vi "MedConfig.vi"(8 "error in (no error)":errorcluster, 11 "Array Parsed Expression":T2[](array[typedef])) -> (0 "error out":errorcluster, 3 "Array Parsed Expression Out":T2[](array[typedef]))   [LabVIEW 2014, in "MathProg.lvlib"]
doc: "Configura las Mediciones."
uses:
  MathProg.lvlib
  TypeDefs/ParsedExpression.ctl
  TypeDefs/typeMed.ctl
panel:
  in  "Resultado:":T1
  out "Tol. Inf. Abs:":sgl
  out "Pre. TI Abs:":sgl
  out "Pre. TS Abs:":sgl
  out "Tol. Sup. Abs:":sgl
  in  "Tol. Inf.:":sgl max=0
  in  "Pre. TI:":sgl max=0
  in  "Pre. TS:":sgl min=0
  in  "Tol. Sup.:":sgl min=0
  in  "Nominal:":sgl
  in  "Description":string caption="Descripción:"
  in  "Stop Med":bool
  in  "Delete Med":bool
  in  "Add Med":bool
  in  "Mediciones":i32(listbox)=-1
  in  "Cancel Med":bool
  in  "Save Med":bool
  in  "Formula:":string
  in  "Edit Med":bool
  out "Medición:":string="M1"
  # "Val Absolutos"
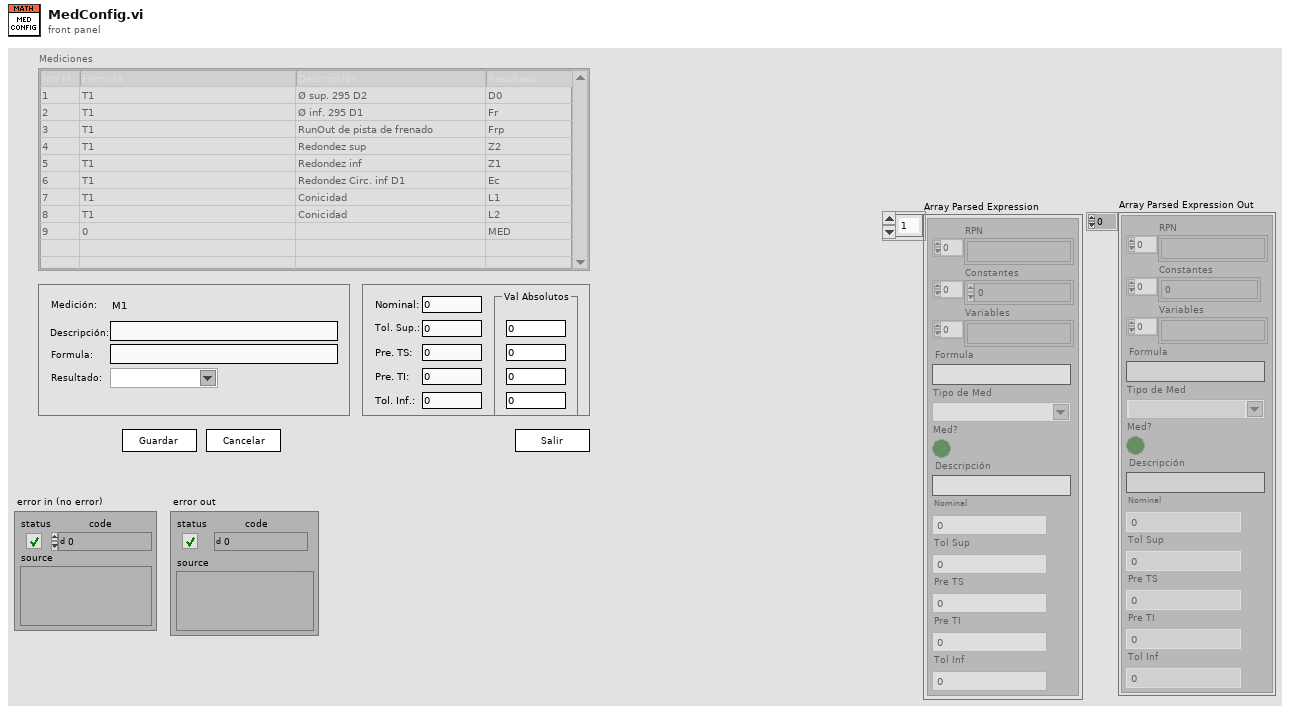
[diagram p1: front panel]
types:
  T1 = typedef "MathProg.lvlib/typeMed.ctl" = string
  T2 = typedef "MathProg.lvlib/ParsedExpression.ctl" = cluster{"RPN ":string[], "Constantes":sgl[], "Variables":string[], "Formula":string, "Tipo de Med":T1, "Med?":bool, "Descripción":string, "Nominal":sgl, "Tol Sup":sgl, "Pre TS":sgl, "Pre TI":sgl, "Tol Inf":sgl}
  T3 = enum8{"Enabled", "Disabled", "Disabled and Grayed Out"}
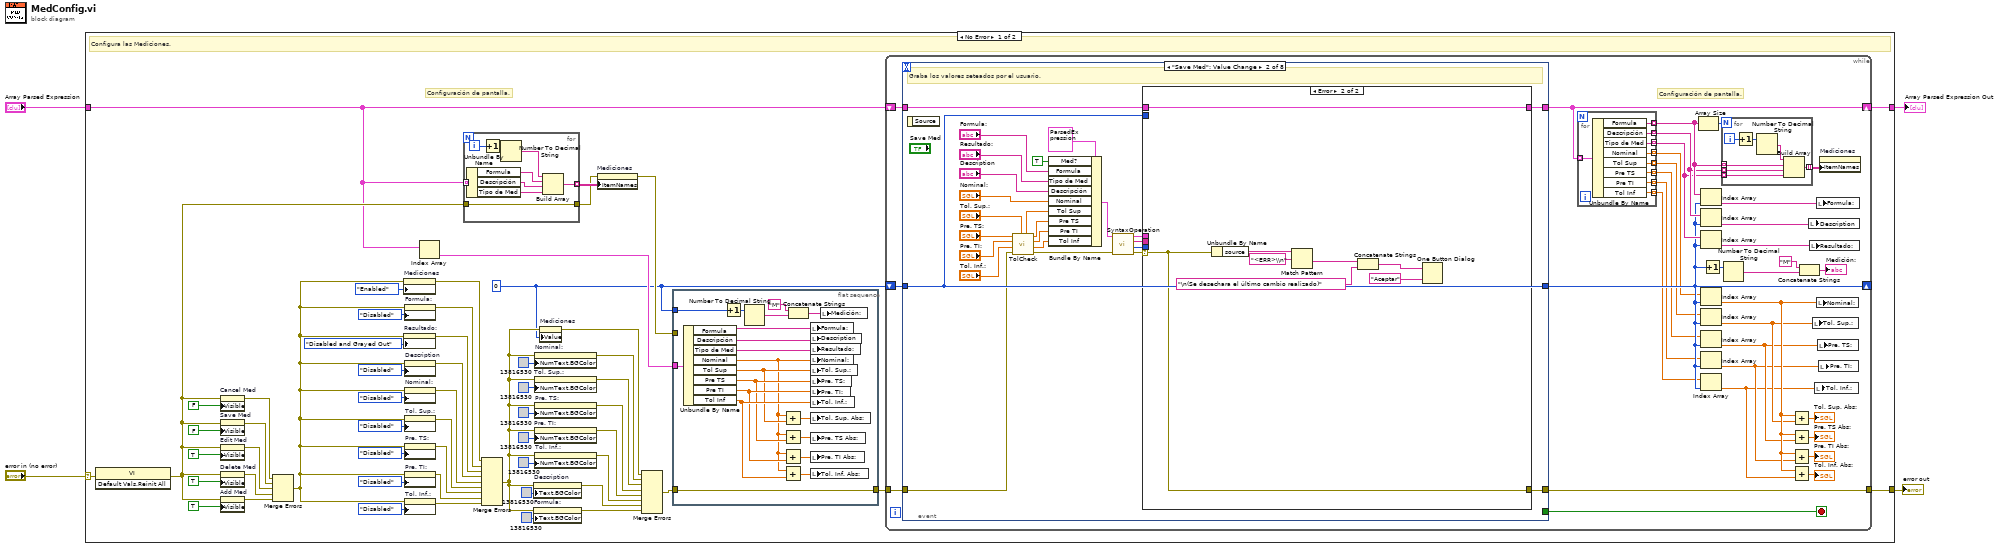
[diagram p0: block diagram]
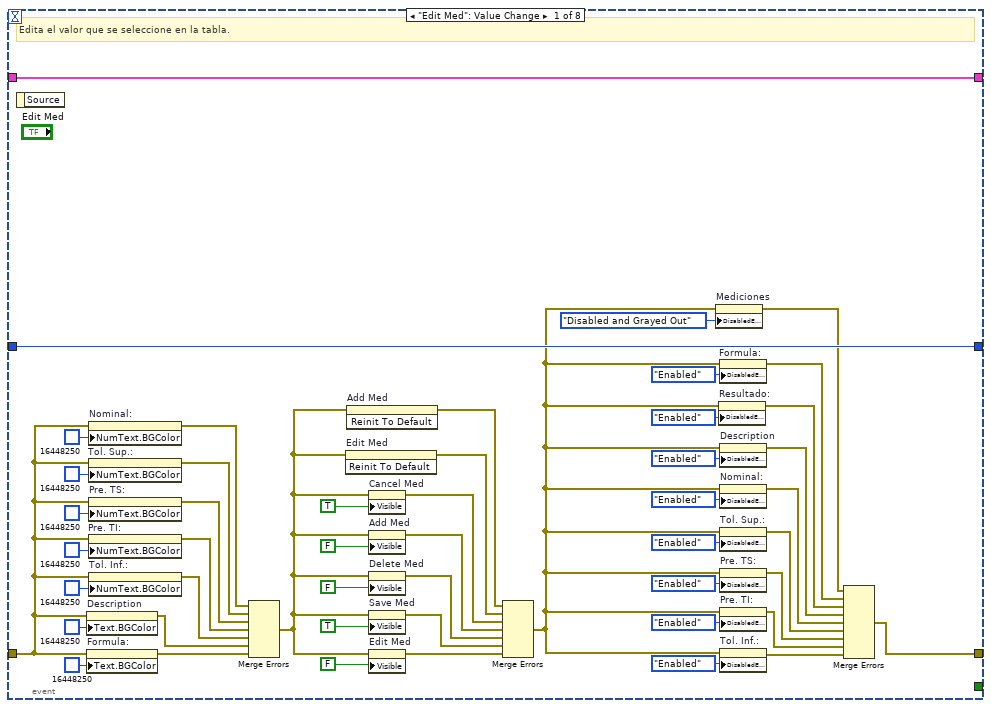
[diagram p2: hidden frame]
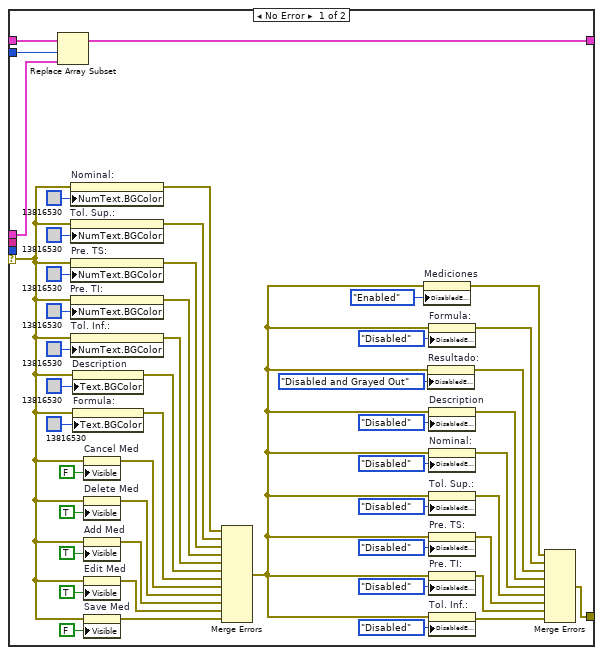
[diagram p3: hidden frame]
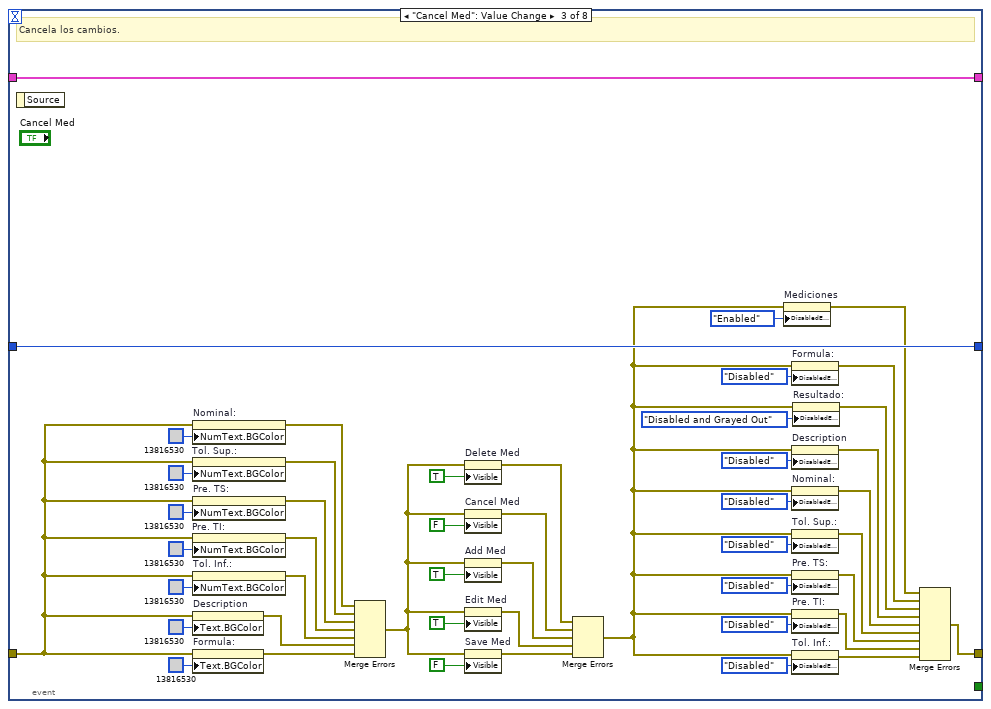
[diagram p4: hidden frame]
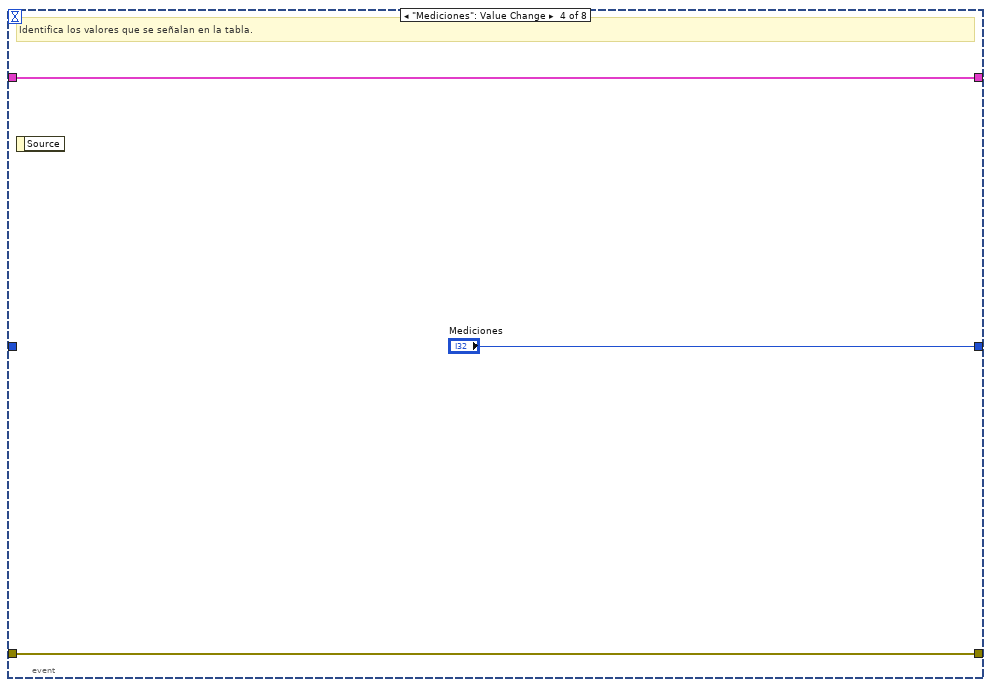
[diagram p5: hidden frame]
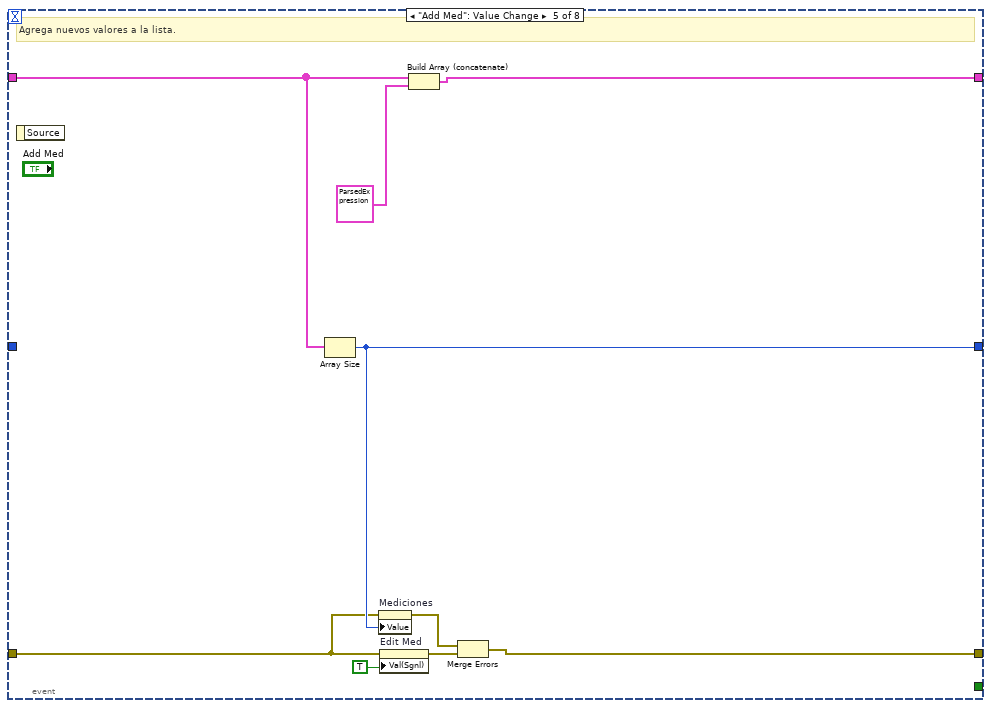
[diagram p6: hidden frame]
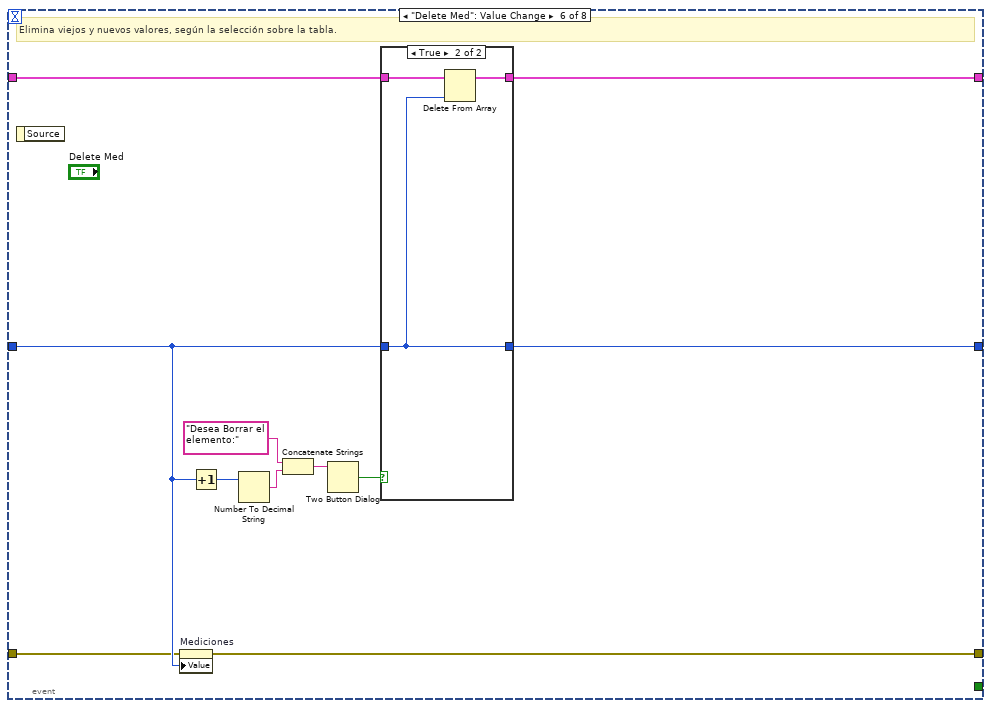
[diagram p7: hidden frame]
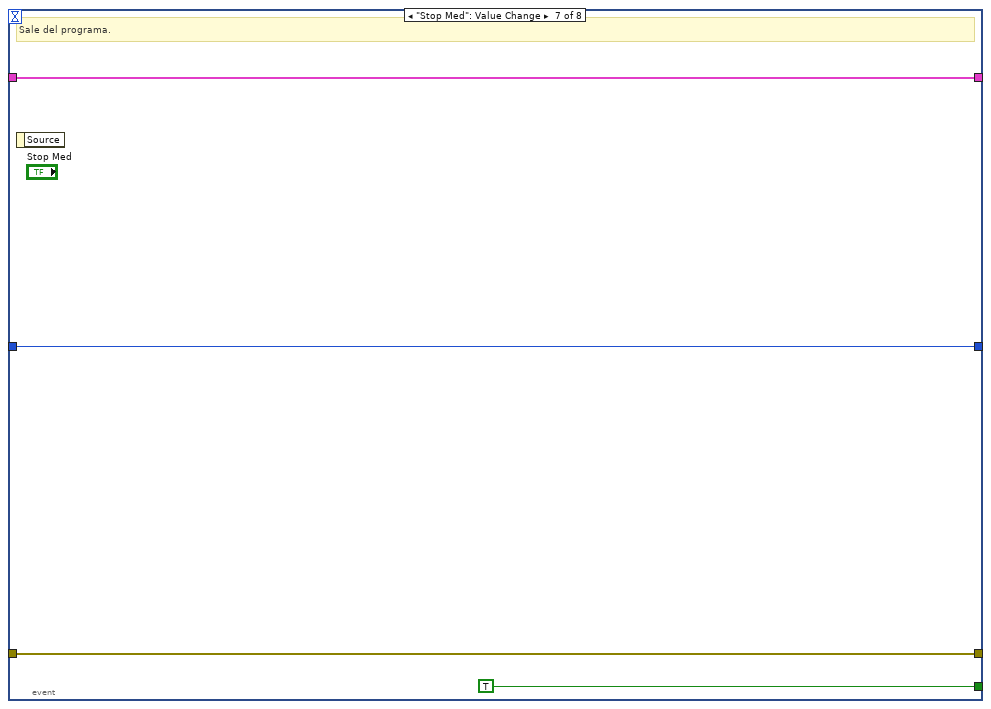
[diagram p9: hidden frame]
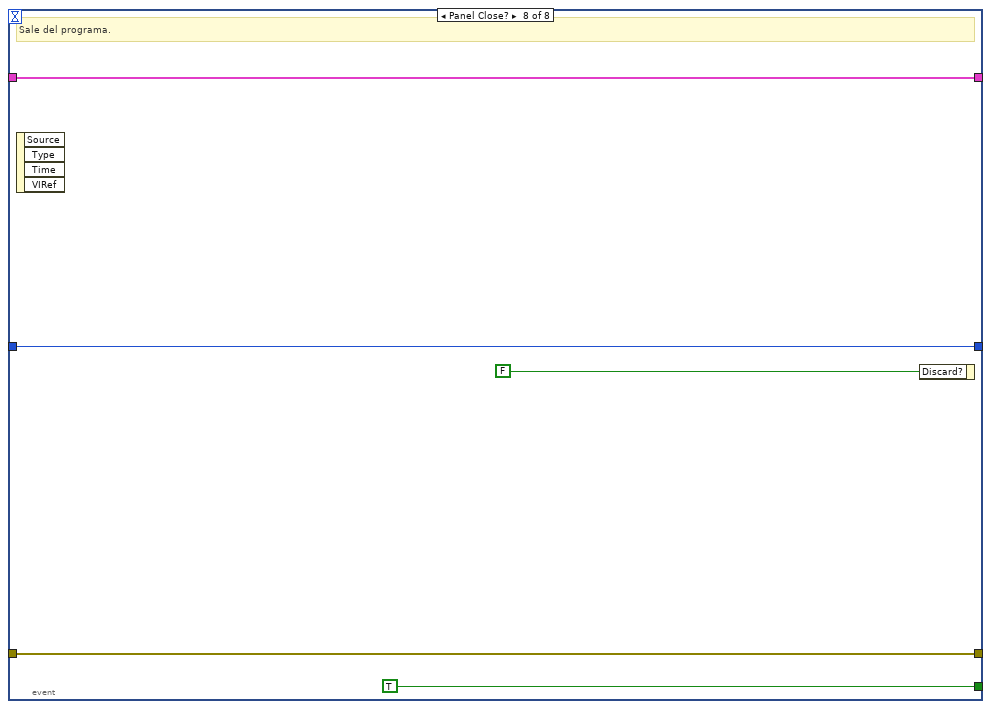
[diagram p10: hidden frame]
diagram:
  n1 = case shown="No Error" "error in (no error)" {
    selector: "error in (no error)" -> [w9 w356]
    tunnel: [w61 w356] -> w4
    tunnel: [w37 w357] -> w3
    tunnel: "Array Parsed Expression" -> [w19 w357]
    frame No Error {
      w12 = 0 ("disabled index (col)")
      # "Configuración de pantalla."
      # "Configura las Mediciones."
      n2 = invoke class="VI" method="Default Vals.Reinit All"(error in=w9) -> (error out=w36:errorcluster)  [unwired: 2 in, 2 out]
      n3 = property on="Cancel Med" class="Bool"(error in=w36, "Visible"=FALSE) -> (error out=w54:errorcluster)  [unwired: 1 in, 1 out]
      n4 = property on="Save Med" class="Bool"(error in=w36, "Visible"=FALSE) -> (error out=w58:errorcluster)  [unwired: 1 in, 1 out]
      n5 = property on="Edit Med" class="Bool (strict)"(error in=w36, "Visible"=TRUE) -> (error out=w57:errorcluster)  [unwired: 1 in, 1 out]
      n6 = property on="Delete Med" class="Bool"(error in=w36, "Visible"=TRUE) -> (error out=w52:errorcluster)  [unwired: 1 in, 1 out]
      n7 = property on="Add Med" class="Bool (strict)"(error in=w36, "Visible"=TRUE) -> (error out=w50:errorcluster)  [unwired: 1 in, 1 out]
      n8 = Merge Errors(w54, w58, w57, w52, w50) -> (w6:errorcluster)
      n9 = property on="Mediciones" class="MCListbox (strict)"(error in=w6, "DisabledEnum"=T3."Enabled" ("Disabled")) -> (error out=w10:errorcluster)  [unwired: 1 in, 1 out]
      n10 = property on="Resultado:" class="CmbBox (strict)"(error in=w6, "DisabledEnum"=T3."Disabled and Grayed Out" ("Disabled")) -> (error out=w7:errorcluster)  [unwired: 1 in, 1 out]
      n11 = property on="Formula:" class="Str"(error in=w6, "DisabledEnum"=T3."Disabled" ("Disabled")) -> (error out=w35:errorcluster)  [unwired: 1 in, 1 out]
      n12 = property on="Description" class="Str"(error in=w6, "DisabledEnum"=T3."Disabled" ("Disabled")) -> (error out=w34:errorcluster)  [unwired: 1 in, 1 out]
      n13 = property on="Nominal:" class="DigNum (strict)"(error in=w6, "DisabledEnum"=T3."Disabled" ("Disabled")) -> (error out=w33:errorcluster)  [unwired: 1 in, 1 out]
      n14 = property on="Tol. Sup.:" class="DigNum (strict)"(error in=w6, "DisabledEnum"=T3."Disabled" ("Disabled")) -> (error out=w32:errorcluster)  [unwired: 1 in, 1 out]
      n15 = property on="Pre. TS:" class="DigNum (strict)"(error in=w6, "DisabledEnum"=T3."Disabled" ("Disabled")) -> (error out=w31:errorcluster)  [unwired: 1 in, 1 out]
      n16 = property on="Pre. TI:" class="DigNum (strict)"(error in=w6, "DisabledEnum"=T3."Disabled" ("Disabled")) -> (error out=w30:errorcluster)  [unwired: 1 in, 1 out]
      n17 = property on="Tol. Inf.:" class="DigNum (strict)"(error in=w6, "DisabledEnum"=T3."Disabled" ("Disabled")) -> (error out=w24:errorcluster)  [unwired: 1 in, 1 out]
      n18 = Index Array(array=w19) -> (element=w18:T2)  [unwired: 1 in]
      n19 = for {
        tunnel: w19 -> [w89] mode=indexing
        tunnel: w36 -> [w81]
        tunnel: [w82] -> w17 mode=indexing
        tunnel: [w81] -> w14
        i -> [w86]
        n20 = Unbundle By Name(w89) -> ("Formula"=w85:string, "Descripción"=w84:string, "Tipo de Med"=w83:T1)
        n21 = Increment(x=w86) -> (x+1=w87:i32)
        n22 = Number To Decimal String(number=w87) -> (decimal integer string=w88:string)  [unwired: 1 in]
        n23 = Build Array(w88, w85, w84, w83) -> (w82:T1[])
      }
      n24 = Merge Errors(w10, w35, w7, w34, w33, w32, w31, w30, w24) -> (w20:errorcluster)
      n25 = property on="Description" class="Str"(error in=w20, "Text.BGColor"=u32 13816530) -> (error out=w21:errorcluster)  [unwired: 1 in, 1 out]
      n26 = property on="Formula:" class="Str"(error in=w20, "Text.BGColor"=u32 13816530) -> (error out=w22:errorcluster)  [unwired: 1 in, 1 out]
      n27 = property on="Nominal:" class="DigNum (strict)"(error in=w20, "NumText.BGColor"=u32 13816530) -> (error out=w39:errorcluster)  [unwired: 1 in, 1 out]
      n28 = property on="Tol. Sup.:" class="DigNum (strict)"(error in=w20, "NumText.BGColor"=u32 13816530) -> (error out=w40:errorcluster)  [unwired: 1 in, 1 out]
      n29 = property on="Pre. TS:" class="DigNum (strict)"(error in=w20, "NumText.BGColor"=u32 13816530) -> (error out=w41:errorcluster)  [unwired: 1 in, 1 out]
      n30 = property on="Pre. TI:" class="DigNum (strict)"(error in=w20, "NumText.BGColor"=u32 13816530) -> (error out=w42:errorcluster)  [unwired: 1 in, 1 out]
      n31 = property on="Tol. Inf.:" class="DigNum (strict)"(error in=w20, "NumText.BGColor"=u32 13816530) -> (error out=w43:errorcluster)  [unwired: 1 in, 1 out]
      n32 = property on="Mediciones" class="MCListbox (strict)"(error in=w20, "Value"=w12) -> (error out=w38:errorcluster)  [unwired: 1 in, 1 out]
      n33 = property on="Mediciones" class="MCListbox (strict)"(error in=w14, "ItemNames"=w17) -> (error out=w15:errorcluster)  [unwired: 1 in, 1 out]
      n34 = Merge Errors(w38, w39, w40, w41, w42, w43, w21, w22) -> (w16:errorcluster)
      n35 = flat-sequence {
        tunnel: w18 -> [w80]
        tunnel: w16 -> [w67]
        tunnel: [w67] -> w13
        tunnel: w15 -> [_]
        tunnel: w12 -> [w62]
        frame #0 {
          n36 = Unbundle By Name(w80) -> ("Formula"=w68:string, "Descripción"=w69:string, "Tipo de Med"=w70:T1, "Nominal"=w71:sgl, "Tol Sup"=w72:sgl, "Pre TS"=w73:sgl, "Pre TI"=w74:sgl, "Tol Inf"=w75:sgl)
          n37 = Increment(x=w62) -> (x+1=w65:i32)
          n38 = Number To Decimal String(number=w65) -> (decimal integer string=w63:string)  [unwired: 1 in]
          n39 = Add(x=w71, y=w72) -> (x+y=w79:sgl)
          n40 = Add(x=w71, y=w73) -> (x+y=w78:sgl)
          n41 = Add(x=w71, y=w74) -> (x+y=w77:sgl)
          n42 = Add(x=w71, y=w75) -> (x+y=w76:sgl)
          n43 = Concatenate Strings("M" ("string"), w63) -> (w66:string)
          n44 = local write "Formula:"(w68) -> ()
          n45 = local write "Description"(w69) -> ()
          n46 = local write "Resultado:"(w70) -> ()
          n47 = local write "Nominal:"(w71) -> ()
          n48 = local write "Tol. Sup.:"(w72) -> ()
          n49 = local write "Pre. TS:"(w73) -> ()
          n50 = local write "Pre. TI:"(w74) -> ()
          n51 = local write "Tol. Inf.:"(w75) -> ()
          n52 = local write "Tol. Sup. Abs:"(w79) -> ()
          n53 = local write "Pre. TS Abs:"(w78) -> ()
          n54 = local write "Pre. TI Abs:"(w77) -> ()
          n55 = local write "Tol. Inf. Abs:"(w76) -> ()
          n56 = local write "Medición:"(w66) -> ()
        }
      }
      n57 = while {
        shift-right: [w111] -> w37
        shift-left: w19 -> [w119]
        shift-right: [w104] -> _
        shift-left: w12 -> [w118]
        tunnel: w13 -> [w122]
        tunnel: [w121] -> w61
        stop <- w120 stop-if-true
        # "Configuración de pantalla."
        n58 = event shown="[1] \"Save Med\": Value Change" {
          selector: _ -> [_ _ _ _ _ _ _ _]
          dyn-events: _ -> [_ _ _ _ _ _ _ _]
          timeout: _ -> [_ _ _ _ _ _ _ _]
          tunnel: w119 -> [w184 w212 w318 w321 w328 w339 w349 w355]
          tunnel: [w184 w211 w318 w321 w330 w338 w349 w355] -> w111
          tunnel: [w183 w213 w317 "Mediciones" w327 w340 w348 w354] -> w104
          tunnel: w118 -> [w183 w213 w317 _ _ w333 w348 w354]
          tunnel: w122 -> [w162 w197 w297 w319 w324 w332 w350 w352]
          tunnel: [w145 w204 w276 w319 w323 w331 w350 w352] -> w121
          tunnel: [_ _ _ _ _ _ TRUE ("Stop Med") TRUE ("Stop Med")] -> w120
          event "Edit Med": Value Change {
            # "Edita el valor que se seleccione en la tabla."
            n59 = event-data() -> ()  [unwired: 1 in, 1 out]
            n60 = property on="Description" class="Str"(error in=w162, "Text.BGColor"=u32 16448250) -> (error out=w160:errorcluster)  [unwired: 1 in, 1 out]
            n61 = property on="Formula:" class="Str"(error in=w162, "Text.BGColor"=u32 16448250) -> (error out=w159:errorcluster)  [unwired: 1 in, 1 out]
            n62 = property on="Nominal:" class="DigNum (strict)"(error in=w162, "NumText.BGColor"=u32 16448250) -> (error out=w174:errorcluster)  [unwired: 1 in, 1 out]
            n63 = property on="Tol. Sup.:" class="DigNum (strict)"(error in=w162, "NumText.BGColor"=u32 16448250) -> (error out=w173:errorcluster)  [unwired: 1 in, 1 out]
            n64 = property on="Pre. TS:" class="DigNum (strict)"(error in=w162, "NumText.BGColor"=u32 16448250) -> (error out=w172:errorcluster)  [unwired: 1 in, 1 out]
            n65 = property on="Pre. TI:" class="DigNum (strict)"(error in=w162, "NumText.BGColor"=u32 16448250) -> (error out=w171:errorcluster)  [unwired: 1 in, 1 out]
            n66 = property on="Tol. Inf.:" class="DigNum (strict)"(error in=w162, "NumText.BGColor"=u32 16448250) -> (error out=w170:errorcluster)  [unwired: 1 in, 1 out]
            n67 = Merge Errors(w174, w173, w172, w171, w170, w160, w159) -> (w161:errorcluster)
            n68 = invoke on="Edit Med" class="Bool (strict)" method="Reinit To Default"(error in=w161) -> (error out=w176:errorcluster)  [unwired: 2 in, 2 out]
            n69 = invoke on="Add Med" class="Bool (strict)" method="Reinit To Default"(error in=w161) -> (error out=w175:errorcluster)  [unwired: 2 in, 2 out]
            n70 = property on="Cancel Med" class="Bool"(error in=w161, "Visible"=TRUE) -> (error out=w177:errorcluster)  [unwired: 1 in, 1 out]
            n71 = property on="Add Med" class="Bool (strict)"(error in=w161, "Visible"=FALSE) -> (error out=w179:errorcluster)  [unwired: 1 in, 1 out]
            n72 = property on="Delete Med" class="Bool"(error in=w161, "Visible"=FALSE) -> (error out=w181:errorcluster)  [unwired: 1 in, 1 out]
            n73 = property on="Save Med" class="Bool"(error in=w161, "Visible"=TRUE) -> (error out=w185:errorcluster)  [unwired: 1 in, 1 out]
            n74 = property on="Edit Med" class="Bool (strict)"(error in=w161, "Visible"=FALSE) -> (error out=w188:errorcluster)  [unwired: 1 in, 1 out]
            n75 = Merge Errors(w175, w176, w177, w179, w181, w185, w188) -> (w140:errorcluster)
            n76 = property on="Mediciones" class="MCListbox (strict)"(error in=w140, "DisabledEnum"=T3."Disabled and Grayed Out" ("Disabled")) -> (error out=w143:errorcluster)  [unwired: 1 in, 1 out]
            n77 = property on="Resultado:" class="CmbBox (strict)"(error in=w140, "DisabledEnum"=T3."Enabled" ("Disabled")) -> (error out=w141:errorcluster)  [unwired: 1 in, 1 out]
            n78 = property on="Formula:" class="Str"(error in=w140, "DisabledEnum"=T3."Enabled" ("Disabled")) -> (error out=w144:errorcluster)  [unwired: 1 in, 1 out]
            n79 = property on="Description" class="Str"(error in=w140, "DisabledEnum"=T3."Enabled" ("Disabled")) -> (error out=w146:errorcluster)  [unwired: 1 in, 1 out]
            n80 = property on="Nominal:" class="DigNum (strict)"(error in=w140, "DisabledEnum"=T3."Enabled" ("Disabled")) -> (error out=w147:errorcluster)  [unwired: 1 in, 1 out]
            n81 = property on="Tol. Sup.:" class="DigNum (strict)"(error in=w140, "DisabledEnum"=T3."Enabled" ("Disabled")) -> (error out=w148:errorcluster)  [unwired: 1 in, 1 out]
            n82 = property on="Pre. TS:" class="DigNum (strict)"(error in=w140, "DisabledEnum"=T3."Enabled" ("Disabled")) -> (error out=w149:errorcluster)  [unwired: 1 in, 1 out]
            n83 = property on="Pre. TI:" class="DigNum (strict)"(error in=w140, "DisabledEnum"=T3."Enabled" ("Disabled")) -> (error out=w150:errorcluster)  [unwired: 1 in, 1 out]
            n84 = property on="Tol. Inf.:" class="DigNum (strict)"(error in=w140, "DisabledEnum"=T3."Enabled" ("Disabled")) -> (error out=w157:errorcluster)  [unwired: 1 in, 1 out]
            n85 = Merge Errors(w143, w144, w141, w146, w147, w148, w149, w150, w157) -> (w145:errorcluster)
          }
          event "Save Med": Value Change {
            # "Graba los valores seteados por el usuario."
            n86 = event-data() -> ()  [unwired: 1 in, 1 out]
            n87 = call "TolCheck.vi"("Tol. Sup.:"="Tol. Sup.:", "error in (no error)"=w197, "Tol. Inf.:"="Tol. Inf.:", "Pre. TI:"="Pre. TI:", "Pre. TS:"="Pre. TS:") -> ("error out"=w196:errorcluster, "Tol. Inf.:"=w193:sgl, "Pre. TI:"=w194:sgl, "Pre. TS:"=w195:sgl, "Tol. Sup.:"=w201:sgl)  [unwired: 2 in]
            n88 = Bundle By Name(cluster=T2 {"RPN "=[], "Constantes"=[], "Variables"=[], "Formula"="", "Tipo de Med"="", "Med?"=FALSE, "Descripción"="", "Nominal"=0.0, "Tol Sup"=0.0, "Pre TS"=0.0, "Pre TI"=0.0, "Tol Inf"=0.0} ("Parsed Expression"), "Med?"=TRUE, "Formula"="Formula:", "Tipo de Med"="Resultado:", "Descripción"="Description", "Nominal"="Nominal:", "Tol Sup"=w201, "Pre TS"=w195, "Pre TI"=w194, "Tol Inf"=w193) -> (w209:T2)
            n89 = call "SyntaxOperation.vi"("error in (no error)"=w196, "Parsed Expression In"=w209) -> ("error out"=w210:errorcluster, "Error Index Out"=w207:i32, "Token"=w190:string[], "Parsed Expression Out"=w205:T2)  [unwired: 6 in]
            n90 = case shown="Error" w210 {
              selector: w210 -> [w241 w269]
              tunnel: w213 -> [w262 _]
              tunnel: w212 -> [w261 w270]
              tunnel: [w260 w270] -> w211
              tunnel: w207 -> [_ _]
              tunnel: w205 -> [w240 _]
              tunnel: [w232 w269] -> w204
              tunnel: w190 -> [_ _]
              frame No Error {
                n91 = Replace Array Subset(array=w261, new element=w240, index=w262) -> (w260:T2[])
                n92 = property on="Nominal:" class="DigNum (strict)"(error in=w241, "NumText.BGColor"=u32 13816530) -> (error out=w233:errorcluster)  [unwired: 1 in, 1 out]
                n93 = property on="Tol. Sup.:" class="DigNum (strict)"(error in=w241, "NumText.BGColor"=u32 13816530) -> (error out=w234:errorcluster)  [unwired: 1 in, 1 out]
                n94 = property on="Pre. TS:" class="DigNum (strict)"(error in=w241, "NumText.BGColor"=u32 13816530) -> (error out=w235:errorcluster)  [unwired: 1 in, 1 out]
                n95 = property on="Pre. TI:" class="DigNum (strict)"(error in=w241, "NumText.BGColor"=u32 13816530) -> (error out=w236:errorcluster)  [unwired: 1 in, 1 out]
                n96 = property on="Tol. Inf.:" class="DigNum (strict)"(error in=w241, "NumText.BGColor"=u32 13816530) -> (error out=w237:errorcluster)  [unwired: 1 in, 1 out]
                n97 = property on="Description" class="Str"(error in=w241, "Text.BGColor"=u32 13816530) -> (error out=w238:errorcluster)  [unwired: 1 in, 1 out]
                n98 = property on="Formula:" class="Str"(error in=w241, "Text.BGColor"=u32 13816530) -> (error out=w239:errorcluster)  [unwired: 1 in, 1 out]
                n99 = property on="Cancel Med" class="Bool"(error in=w241, "Visible"=FALSE) -> (error out=w258:errorcluster)  [unwired: 1 in, 1 out]
                n100 = property on="Delete Med" class="Bool"(error in=w241, "Visible"=TRUE) -> (error out=w259:errorcluster)  [unwired: 1 in, 1 out]
                n101 = property on="Add Med" class="Bool (strict)"(error in=w241, "Visible"=TRUE) -> (error out=w255:errorcluster)  [unwired: 1 in, 1 out]
                n102 = property on="Edit Med" class="Bool (strict)"(error in=w241, "Visible"=TRUE) -> (error out=w250:errorcluster)  [unwired: 1 in, 1 out]
                n103 = property on="Save Med" class="Bool"(error in=w241, "Visible"=FALSE) -> (error out=w251:errorcluster)  [unwired: 1 in, 1 out]
                n104 = Merge Errors(w233, w234, w235, w236, w237, w238, w239, w258, w259, w255, w250, w251) -> (w215:errorcluster)
                n105 = property on="Mediciones" class="MCListbox (strict)"(error in=w215, "DisabledEnum"=T3."Enabled" ("Disabled")) -> (error out=w217:errorcluster)  [unwired: 1 in, 1 out]
                n106 = property on="Resultado:" class="CmbBox (strict)"(error in=w215, "DisabledEnum"=T3."Disabled and Grayed Out" ("Disabled")) -> (error out=w216:errorcluster)  [unwired: 1 in, 1 out]
                n107 = property on="Formula:" class="Str"(error in=w215, "DisabledEnum"=T3."Disabled" ("Disabled")) -> (error out=w219:errorcluster)  [unwired: 1 in, 1 out]
                n108 = property on="Description" class="Str"(error in=w215, "DisabledEnum"=T3."Disabled" ("Disabled")) -> (error out=w220:errorcluster)  [unwired: 1 in, 1 out]
                n109 = property on="Nominal:" class="DigNum (strict)"(error in=w215, "DisabledEnum"=T3."Disabled" ("Disabled")) -> (error out=w221:errorcluster)  [unwired: 1 in, 1 out]
                n110 = property on="Tol. Sup.:" class="DigNum (strict)"(error in=w215, "DisabledEnum"=T3."Disabled" ("Disabled")) -> (error out=w222:errorcluster)  [unwired: 1 in, 1 out]
                n111 = property on="Pre. TS:" class="DigNum (strict)"(error in=w215, "DisabledEnum"=T3."Disabled" ("Disabled")) -> (error out=w223:errorcluster)  [unwired: 1 in, 1 out]
                n112 = property on="Pre. TI:" class="DigNum (strict)"(error in=w215, "DisabledEnum"=T3."Disabled" ("Disabled")) -> (error out=w224:errorcluster)  [unwired: 1 in, 1 out]
                n113 = property on="Tol. Inf.:" class="DigNum (strict)"(error in=w215, "DisabledEnum"=T3."Disabled" ("Disabled")) -> (error out=w231:errorcluster)  [unwired: 1 in, 1 out]
                n114 = Merge Errors(w217, w219, w216, w220, w221, w222, w223, w224, w231) -> (w232:errorcluster)
              }
              frame Error {
                n115 = Unbundle By Name(w269) -> ("source"=w267:string)
                n116 = Match Pattern(string=w267, regular expression="<ERR>\\n") -> (after substring=w265:string)  [unwired: 1 in, 3 out]
                n117 = Concatenate Strings(w265, "\n(Se desechara el último cambio realizado)" ("button name (\"OK\")")) -> (w263:string)
                n118 = One Button Dialog(message=w263, button name ("OK")="Aceptar") -> ()  [unwired: 1 out]
              }
            }
          }
          event "Cancel Med": Value Change {
            # "Cancela los cambios."
            n119 = event-data() -> ()  [unwired: 1 in, 1 out]
            n120 = property on="Nominal:" class="DigNum (strict)"(error in=w297, "NumText.BGColor"=u32 13816530) -> (error out=w291:errorcluster)  [unwired: 1 in, 1 out]
            n121 = property on="Tol. Sup.:" class="DigNum (strict)"(error in=w297, "NumText.BGColor"=u32 13816530) -> (error out=w292:errorcluster)  [unwired: 1 in, 1 out]
            n122 = property on="Pre. TS:" class="DigNum (strict)"(error in=w297, "NumText.BGColor"=u32 13816530) -> (error out=w293:errorcluster)  [unwired: 1 in, 1 out]
            n123 = property on="Pre. TI:" class="DigNum (strict)"(error in=w297, "NumText.BGColor"=u32 13816530) -> (error out=w294:errorcluster)  [unwired: 1 in, 1 out]
            n124 = property on="Tol. Inf.:" class="DigNum (strict)"(error in=w297, "NumText.BGColor"=u32 13816530) -> (error out=w295:errorcluster)  [unwired: 1 in, 1 out]
            n125 = property on="Description" class="Str"(error in=w297, "Text.BGColor"=u32 13816530) -> (error out=w301:errorcluster)  [unwired: 1 in, 1 out]
            n126 = property on="Formula:" class="Str"(error in=w297, "Text.BGColor"=u32 13816530) -> (error out=w300:errorcluster)  [unwired: 1 in, 1 out]
            n127 = Merge Errors(w291, w292, w293, w294, w295, w301, w300) -> (w296:errorcluster)
            n128 = property on="Delete Med" class="Bool"(error in=w296, "Visible"=TRUE) -> (error out=w308:errorcluster)  [unwired: 1 in, 1 out]
            n129 = property on="Cancel Med" class="Bool"(error in=w296, "Visible"=FALSE) -> (error out=w307:errorcluster)  [unwired: 1 in, 1 out]
            n130 = property on="Add Med" class="Bool (strict)"(error in=w296, "Visible"=TRUE) -> (error out=w311:errorcluster)  [unwired: 1 in, 1 out]
            n131 = property on="Edit Med" class="Bool (strict)"(error in=w296, "Visible"=TRUE) -> (error out=w316:errorcluster)  [unwired: 1 in, 1 out]
            n132 = property on="Save Med" class="Bool"(error in=w296, "Visible"=FALSE) -> (error out=w315:errorcluster)  [unwired: 1 in, 1 out]
            n133 = Merge Errors(w308, w307, w311, w316, w315) -> (w272:errorcluster)
            n134 = property on="Mediciones" class="MCListbox (strict)"(error in=w272, "DisabledEnum"=T3."Enabled" ("Disabled")) -> (error out=w274:errorcluster)  [unwired: 1 in, 1 out]
            n135 = property on="Formula:" class="Str"(error in=w272, "DisabledEnum"=T3."Disabled" ("Disabled")) -> (error out=w277:errorcluster)  [unwired: 1 in, 1 out]
            n136 = property on="Description" class="Str"(error in=w272, "DisabledEnum"=T3."Disabled" ("Disabled")) -> (error out=w278:errorcluster)  [unwired: 1 in, 1 out]
            n137 = property on="Nominal:" class="DigNum (strict)"(error in=w272, "DisabledEnum"=T3."Disabled" ("Disabled")) -> (error out=w279:errorcluster)  [unwired: 1 in, 1 out]
            n138 = property on="Tol. Sup.:" class="DigNum (strict)"(error in=w272, "DisabledEnum"=T3."Disabled" ("Disabled")) -> (error out=w280:errorcluster)  [unwired: 1 in, 1 out]
            n139 = property on="Pre. TS:" class="DigNum (strict)"(error in=w272, "DisabledEnum"=T3."Disabled" ("Disabled")) -> (error out=w281:errorcluster)  [unwired: 1 in, 1 out]
            n140 = property on="Pre. TI:" class="DigNum (strict)"(error in=w272, "DisabledEnum"=T3."Disabled" ("Disabled")) -> (error out=w282:errorcluster)  [unwired: 1 in, 1 out]
            n141 = property on="Tol. Inf.:" class="DigNum (strict)"(error in=w272, "DisabledEnum"=T3."Disabled" ("Disabled")) -> (error out=w289:errorcluster)  [unwired: 1 in, 1 out]
            n142 = property on="Resultado:" class="CmbBox (strict)"(error in=w272, "DisabledEnum"=T3."Disabled and Grayed Out" ("Disabled")) -> (error out=w271:errorcluster)  [unwired: 1 in, 1 out]
            n143 = Merge Errors(w274, w277, w271, w278, w279, w280, w281, w282, w289) -> (w276:errorcluster)
          }
          event "Mediciones": Value Change {
            # "Identifica los valores que se señalan en la tabla."
            n144 = event-data() -> ()  [unwired: 1 in, 1 out]
          }
          event "Add Med": Value Change {
            # "Agrega nuevos valores a la lista."
            n145 = event-data() -> ()  [unwired: 1 in, 1 out]
            n146 = Array Size(array=w328) -> (size(s)=w327:i32)
            n147 = property on="Mediciones" class="MCListbox (strict)"(error in=w324, "Value"=w327) -> (error out=w326:errorcluster)  [unwired: 1 in, 1 out]
            n148 = property on="Edit Med" class="Bool (strict)"(error in=w324, "Val(Sgnl)"=TRUE) -> (error out=w325:errorcluster)  [unwired: 1 in, 1 out]
            n149 = Build Array (concatenate)(w328, T2 {"RPN "=[" "], "Constantes"=[0.0], "Variables"=[" "], "Formula"="0 ", "Tipo de Med"="MED", "Med?"=TRUE, "Descripción"=" ", "Nominal"=0.0, "Tol Sup"=0.0, "Pre TS"=0.0, "Pre TI"=0.0, "Tol Inf"=0.0} ("Parsed Expression In")) -> (w330:T2[])
            n150 = Merge Errors(w326, w325) -> (w323:errorcluster)
          }
          event "Delete Med": Value Change {
            # "Elimina viejos y nuevos valores, según la selección sobre la tabla."
            n151 = event-data() -> ()  [unwired: 1 in, 1 out]
            n152 = property on="Mediciones" class="MCListbox (strict)"(error in=w332, "Value"=w333) -> (error out=w331:errorcluster)  [unwired: 1 in, 1 out]
            n153 = Increment(x=w333) -> (x+1=w334:i32)
            n154 = Number To Decimal String(number=w334) -> (decimal integer string=w336:string)  [unwired: 1 in]
            n155 = Concatenate Strings("Desea Borrar el elemento:" ("message"), w336) -> (w335:string)
            n156 = Two Button Dialog(message=w335) -> (T button?=w341:bool)  [unwired: 2 in]
            n157 = case shown="True" w341 {
              tunnel: w339 -> [w342 w346]
              tunnel: [w343 w344] -> w340
              tunnel: w333 -> [w343 w344]
              tunnel: [w342 w345] -> w338
              frame False {
              }
              frame True {
                n158 = Delete From Array(array=w346, index=w344) -> (array with subset deleted=w345:T2[])  [unwired: 1 in, 1 out]
              }
            }
          }
          event "Stop Med": Value Change {
            # "Sale del programa."
            n159 = event-data() -> ()  [unwired: 1 in, 1 out]
          }
          event Panel Close? {
            # "Sale del programa."
            n160 = event-data() -> ()  [unwired: 1 in, 4 out]
            n161 = event-data("Discard?"=FALSE) -> ()  [unwired: 1 in, 1 out]
          }
        }
        n162 = for {
          tunnel: w111 -> [w131] mode=indexing
          tunnel: [w130] -> w110 mode=indexing
          tunnel: [w129] -> w108 mode=indexing
          tunnel: [w128] -> w105 mode=indexing
          tunnel: [w127] -> w99 mode=indexing
          tunnel: [w126] -> w100 mode=indexing
          tunnel: [w125] -> w101 mode=indexing
          tunnel: [w124] -> w102 mode=indexing
          tunnel: [w123] -> w103 mode=indexing
          n163 = Unbundle By Name(w131) -> ("Formula"=w130:string, "Descripción"=w129:string, "Tipo de Med"=w128:T1, "Nominal"=w127:sgl, "Tol Sup"=w126:sgl, "Pre TS"=w125:sgl, "Pre TI"=w124:sgl, "Tol Inf"=w123:sgl)
        }
        n164 = Array Size(array=w110) -> (size(s)=w112:i32)
        n165 = Index Array(array=w110, index=w104) -> (element=w114:string)
        n166 = Index Array(array=w108, index=w104) -> (element=w109:string)
        n167 = Index Array(array=w105, index=w104) -> (element=w107:T1)
        n168 = Index Array(array=w99, index=w104) -> (element=w94:sgl)
        n169 = Index Array(array=w100, index=w104) -> (element=w93:sgl)
        n170 = Index Array(array=w101, index=w104) -> (element=w92:sgl)
        n171 = Index Array(array=w102, index=w104) -> (element=w91:sgl)
        n172 = Index Array(array=w103, index=w104) -> (element=w90:sgl)
        n173 = Increment(x=w104) -> (x+1=w106:i32)
        n174 = for {
          N: w112 -> [_]
          tunnel: w110 -> [w138] mode=indexing
          tunnel: [w136] -> w113 mode=indexing
          tunnel: w108 -> [w133] mode=indexing
          tunnel: w105 -> [w132] mode=indexing
          i -> [w134]
          n175 = Increment(x=w134) -> (x+1=w135:i32)
          n176 = Number To Decimal String(number=w135) -> (decimal integer string=w137:string)  [unwired: 1 in]
          n177 = Build Array(w137, w138, w133, w132) -> (w136:T1[])
        }
        n178 = Number To Decimal String(number=w106) -> (decimal integer string=w117:string)  [unwired: 1 in]
        n179 = Add(x=w94, y=w93) -> (x+y=→"Tol. Sup. Abs:":sgl)
        n180 = Add(x=w94, y=w92) -> (x+y=→"Pre. TS Abs:":sgl)
        n181 = Add(x=w94, y=w91) -> (x+y=→"Pre. TI Abs:":sgl)
        n182 = Add(x=w94, y=w90) -> (x+y=→"Tol. Inf. Abs:":sgl)
        n183 = Concatenate Strings("M" ("string"), w117) -> (→"Medición:":string)
        n184 = local write "Description"(w109) -> ()
        n185 = local write "Resultado:"(w107) -> ()
        n186 = local write "Tol. Sup.:"(w93) -> ()
        n187 = local write "Tol. Inf.:"(w90) -> ()
        n188 = local write "Formula:"(w114) -> ()
        n189 = local write "Nominal:"(w94) -> ()
        n190 = local write "Pre. TS:"(w92) -> ()
        n191 = local write "Pre. TI:"(w91) -> ()
        n192 = property on="Mediciones" class="MCListbox (strict)"("ItemNames"=w113) -> ()  [unwired: 2 in, 2 out]
      }
    }
    frame Error {
    }
  }
  "error out" <- w4
  "Array Parsed Expression Out" <- w3
